vi "Create Front Panel Events.vi"(8 "error in (no error)":errorcluster, 11 "Splash Screen in":refnum<class "Splash Screen.lvclass">) -> (0 "error out":errorcluster, 3 "Splash Screen out":refnum<class "Splash Screen.lvclass">)   [LabVIEW 2015, in "Splash Screen.lvlib" / "Splash Screen.lvclass"]
uses:
  Splash Screen.lvclass
  UI Window/UI Window.lvclass
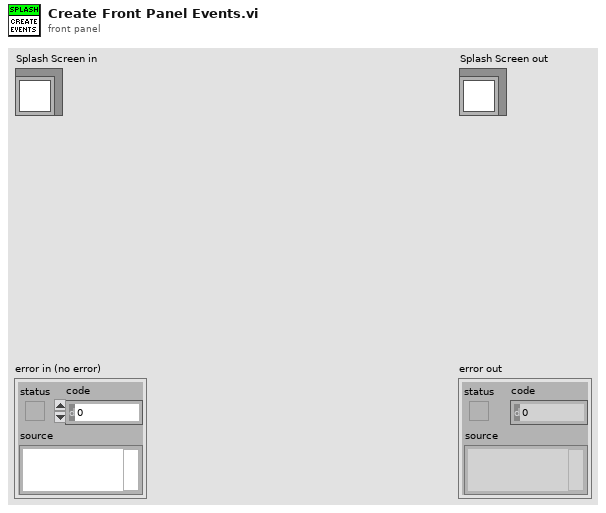
[diagram p1: front panel]
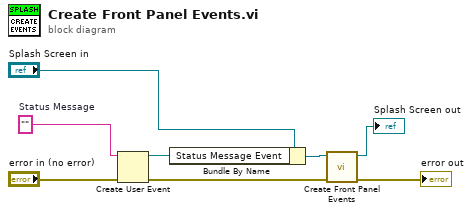
[diagram p0: block diagram]
diagram:
  w5 = ""  # Status Message
  n1 = Create User Event(user event datatype=w5, error in="error in (no error)") -> (user event=w6:refnum<user-event>, error out=w1:errorcluster)
  n2 = Bundle By Name(cluster="Splash Screen in", "Status Message Event"=w6) -> (w3:refnum<class "Splash Screen.lvclass">)
  n3 = call-parent "Create Front Panel Events.vi"("error in (no error)"=w1, "UI Window in"=w3) -> ("error out"=→"error out":errorcluster, "UI Window out"=→"Splash Screen out":refnum<class "Splash Screen.lvclass">)  [unwired: 8 in]
